vi "(SubVI)I2C_Log_Append Header.vi"(5 "Log Ref":refnum<vi>, 10 "error in (no error)":errorcluster caption="에러 입력(에러 없음)", 11 "Header":string) -> (2 "error out":errorcluster caption="에러 출력")   [LabVIEW 2020]
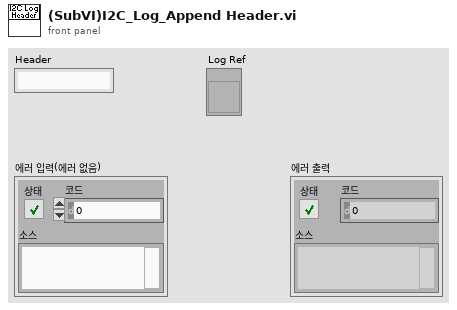
[diagram p1: front panel]
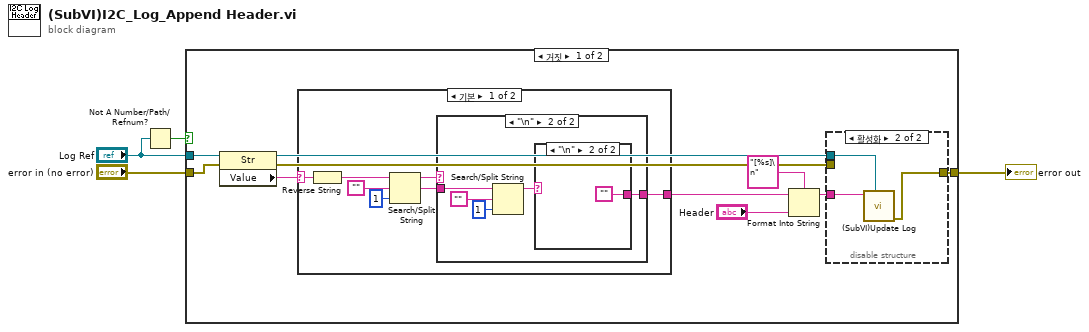
[diagram p0: block diagram]
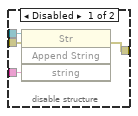
[diagram p2: hidden frame]
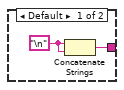
[diagram p3: hidden frame]
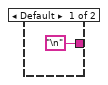
[diagram p4: hidden frame]
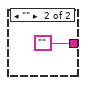
[diagram p5: hidden frame]
diagram:
  n1 = Not A Number/Path/Refnum?(number/path/refnum="Log Ref") -> (NaN/Path/Refnum?=w1:bool)
  n2 = case shown="거짓" w1 {
    tunnel: "Log Ref" -> [w14 _]
    tunnel: "error in (no error)" -> [w6 w39]
    tunnel: [w5 w39] -> w3
    frame False {
      n3 = property class="Str"(reference=w14, error in=w6) -> (reference out=w12:refnum<vi>, error out=w7:errorcluster, "Value"=w13:string)
      n4 = case shown="기본" w13 {
        selector: w13 -> [w28 _]
        tunnel: [w22 ""] -> w11
        frame Default {
          n5 = Reverse String(1:w28) -> (0:w27:string)
          n6 = Search/Split String(string=w27, search string/char (-)="", offset (0)=1 ("오프셋(0)")) -> (substring before match=w24:string, match + rest of string=w23:string)  [unwired: 1 out]
          n7 = case shown="\"\\n\"" w24 {
            tunnel: w23 -> [_ w33]
            tunnel: [w29 w31] -> w22
            frame Default {
              w30 = "\n"
              n8 = Concatenate Strings(w30, w30) -> (w29:string)
            }
            frame "\n" {
              n9 = Search/Split String(string=w33, search string/char (-)="", offset (0)=1 ("오프셋(0)")) -> (substring before match=w32:string)  [unwired: 2 out]
              n10 = case shown="\"\\n\"" w32 {
                tunnel: ["\n" ""] -> w31
                frame Default {
                }
                frame "\n" {
                }
              }
            }
          }
        }
        frame "" {
        }
      }
      n11 = Format Into String(format string="[%s]\n" ("포맷 문자열"), initial string=w11, "Header") -> (resulting string=w8:string)  [unwired: 1 in, 1 out]
      n12 = disable-structure shown="활성화" {
        disable-tunnel: w12 -> [w18 w20]
        disable-tunnel: w8 -> [w17 w21]
        disable-tunnel: w7 -> [w16 _]
        disable-tunnel: [w15 w19] -> w5
        frame Disabled {
          n13 = invoke class="Str" method="Append String"(reference=w18, error in=w16, "string"=w17) -> (error out=w15:errorcluster)  [unwired: 1 in, 3 out]
        }
        frame Enabled {
          n14 = call "(SubVI)Update Log.vi"("Log Ref"=w20, "Log"=w21) -> ("error out"=w19:errorcluster)  [unwired: 8 in, 1 out]
        }
      }
    }
    frame True {
    }
  }
  "error out" <- w3
